vi "KWP Diagnostics Engine.vi"(8 "error in (no error)":errorcluster, 11 "State Variables":T1={"TCP Refs"={"Connection List"=refnum, "listener ID"=refnum}, "Stop"=refnum, "Top VI"=refnum, "Parameters"={"Name"="", "PID Lookup"=variant, "DID Lookup"=variant, "Section Properties"={"CAN"={"Database File"=path "", "CAN Interface"=enum."CAN0", "Baud Rate"=0, "Diagnostic Protocol"=enum."GMLAN", "Transport Protocol"=enum."ISO TP - Normal Mode", "Transmit ID"=0, "Receive ID"=0, "Transmit Extension"=0, "Receive Extension"=0, "Receive UUDT ID"=0, "Enable Stream"=TRUE, "VW TP Channel ID"=0}, "DPIDs"=[], "DTC descriptor"={"DTC Byte Length"=2, "Status Byte Length"=1, "Add Data Byte Length"=1, "Byte Order"=enum."Motorola"}, "PIDs"=[], "DIDs"=[], "CPIDs"=[]}, "ChanRefs"={"ToVS.PIDs"={"Name"="", "Write to VS Engine FIFO"=refnum, "Pairs"={"Refs"=[], "Values"=[]}}, "ToVS.DIDs"={"Name"="", "Write to VS Engine FIFO"=refnum, "Pairs"={"Refs"=[], "Values"=[]}}, "ToVS.DTCs"={"Name"="", "Write to VS Engine FIFO"=refnum, "Pairs"={"Refs"=[], "Values"=[]}}, "ToVS.DTCCount"={"Name"="", "Write to VS Engine FIFO"=refnum, "Pairs"={"Refs"=[], "Values"=[]}}, "ToVS.Success"={"Name"="", "Write to VS Engine FIFO"=refnum, "Pairs"={"Refs"=[], "Values"=[]}}, "FromVS.CPIDs"={"Name"="", "Read from VS Engine FIFO"=refnum, "Pairs"={"Refs"=[], "Values"=[]}}, "Cmds"={"Name"="", "Write to VS Engine FIFO"=refnum, "Read from VS Engine FIFO"=refnum, "Pairs"={"Chan Refs"=[], "Prev. Values"=[]}}}, "CPID Lookup"=variant, "DPID Lookup"=variant}, "ADCS Connection"={"Diag CAN Handle"=0, "Transport Protocol"=enum."ISO TP - Normal Mode", "Receive Address Extension"=0, "Transmit Address Extension"=0, "Receive CAN Id"=0, "Transmit CAN Id"=0, "Diag CAN Queue"=refnum, "Log Frames ?"=FALSE, "My TP Address"=0, "Other TP Address"=0, "T1"=0, "T2"=0, "T3"=0, "T4"=0, "Tx SN"=0, "Block Size"=0, "Rx SN"=0, "VW TP Initialized?"=FALSE, "Tx block no"=0, "baud rate"=0, "Interface"="", "Channel Diag CAN Handle"=0, "UDP Connection ID"=refnum, "TCP Connection ID"=refnum, "Target IP Addr"=0, "Source Address"=0, "Target Address"=0, "Send Header NACK?"=FALSE, "DLL Handle"=0, "NAD"=0, "Time Stamp read first"=0.0, "Time Stamp read last"=0.0, "Time Stamp write first"=0.0, "Time Stamp write last"=0.0, "Time Stamp write"=0.0, "Time Stamp read"=0.0}, "XNET References"={"Database"="", "GMLAN DPID Session"="", "Cluster"=""}, "BufferedCmds"=refnum, "XNETEngine (GMLAN)"=refnum} {"Parameters"."ChanRefs"."Cmds"."Pairs"."Chan Refs" format="%.0x"; "Parameters"."ChanRefs"."ToVS.Success"."Pairs"."Refs" format="%.0x"; "Parameters"."ChanRefs"."ToVS.DTCCount"."Pairs"."Refs" format="%.0x"; "Parameters"."ChanRefs"."ToVS.DTCs"."Pairs"."Refs" format="%.0x"; "Parameters"."ChanRefs"."ToVS.PIDs"."Pairs"."Refs" format="%.0x"; "Parameters"."ChanRefs"."ToVS.DIDs"."Pairs"."Refs" format="%.0x"; "Parameters"."Section Properties"."CPIDs"."Signals"."Byte Order" items=["Little Endian", "Big Endian"]; "Parameters"."Section Properties"."CPIDs"."Signals"."Data Type" items=["Signed", "Unsigned", "IEEE Float"]; "Parameters"."Section Properties"."DIDs"."Signals"."Byte Order" items=["Little Endian", "Big Endian"]; "Parameters"."Section Properties"."DIDs"."Signals"."Data Type" items=["Signed", "Unsigned", "IEEE Float"]; "Parameters"."Section Properties"."CAN"."VW TP Channel ID" format="%.0x"; "Parameters"."Section Properties"."CAN"."Receive UUDT ID" format="%.0x"; "Parameters"."Section Properties"."CAN"."Receive Extension" format="%.0x"; "Parameters"."Section Properties"."CAN"."Transmit Extension" format="%.0x"; "Parameters"."Section Properties"."CAN"."Receive ID" format="%.0x"; "Parameters"."Section Properties"."CAN"."Transmit ID" format="%.0x"; "Parameters"."Section Properties"."PIDs"."Signals"."Byte Order" items=["Little Endian", "Big Endian"]; "Parameters"."Section Properties"."PIDs"."Signals"."Data Type" items=["Signed", "Unsigned", "IEEE Float"]}) -> (0 "error out":errorcluster)   [LabVIEW 2015, in "Diagnostics Addon Engine.lvlib"]
uses:
  Diagnostics Addon Engine.lvlib
  State Variables.ctl
  TCP Refs.ctl
  STM/STM Lookup Table Ref.ctl
  Stop FG/Stop Global Ref.ctl
  Main Configuration.ctl
  Section Properties.ctl
  Shared/CAN Configuration.ctl
  Shared/CAN Interface.ctl
  Shared/Diagnostic Protocols.ctl
  Shared/Transport Protocols.ctl
  Shared/DPID Parameters.ctl
  Shared/DPID Periodic Rate.ctl
  <vilib>/Automotive Diagnostic Command Set/Diagnostic Protocols.llb/DTC Descriptor.ctl
  Shared/DIDPID Parameters.ctl
  Shared/DIDPID Signal Parameters.ctl
  VS Data Channels.ctl
  Inline Async API/Controls/Write To VS Engine.ctl
  <vilib>/NI Veristand/Custom Device API/Data Reference.ctl
  Inline Async API/Controls/Read From VS Engine.ctl
  <vilib>/NI Veristand/Custom Device API/Block Data Reference.ctl
  Inline Async API/Controls/ReadWrite Data.ctl
  <vilib>/Automotive Diagnostic Command Set/Diagnostic Transport.llb/Diag Reference.ctl
  <vilib>/Automotive Diagnostic Command Set/Diagnostic Transport.llb/Transport Protocol Selector.ctl
  <vilib>/Automotive Diagnostic Command Set/Diagnostic Transport.llb/Diag CAN Frame Log.ctl
  XNET References.ctl
  <vilib>/NI/AMC/Message Queue.ctl
  <vilib>/NI/AMC/Message.ctl
  <vilib>/NI/Tools/Keyed Array/KeyedArray.ctl
  Stop FG/Stop Global Commands.ctl
  Shared/DTC and Timestamp Cluster.ctl
  Datatable Lookup Positions.ctl
  <vilib>/NI/AMC/Create Single Message.vi
  <vilib>/NI/AMC/Update Message Routing Info.vi
  <vilib>/NI/Tools/Keyed Array/Map String.vi
  <vilib>/NI/AMC/Read Termination Message.vi
  <vilib>/NI/Tools/String/Get Case Matching.vi
  <vilib>/xnet/xnet.llb/XNET Convert (Frame Raw to Signal).vi
  Convert ID to Raw Data.vi
  Shared/GUID Lookup.vi
  <vilib>/NI/AMC/Send Message.vi
  <vilib>/NI/AMC/Globals.vi
  Stop FG/Stop FG.lvlib
  Error Handling API/Error Handling API.lvlib
  <vilib>/NI Veristand/Custom Device Tools/Custom Device Utility Library/Custom Device Utility Library.lvlib
  Shared/Diagnostics Addon Shared.lvlib
  <vilib>/NI/AMC/AMC.lvlib
  <vilib>/NI/Tools/Keyed Array/Tools_KeyedArray.lvlib
  <vilib>/NI Veristand/Custom Device API/Custom Device API.lvlib
  <vilib>/addons/Automotive Diagnostic Command Set/NI_Automotive Diagnostic Command Set.lvlib
  Inline Async API/Inline Async API.lvlib
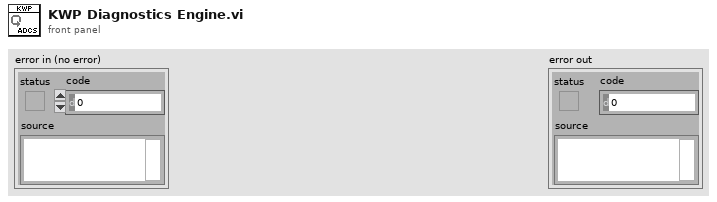
[diagram p1: front panel]
types:
  T1 = typedef "Diagnostics Addon Engine.lvlib/State Variables.ctl" = cluster{"TCP Refs":T2, "Stop":T4, "Top VI":refnum<vi>, "Parameters":T5, "ADCS Connection":T22, "XNET References":T24, "BufferedCmds":T25, "XNETEngine (GMLAN)":T25}
  T2 = typedef "Diagnostics Addon Engine.lvlib/TCP Refs.ctl" = cluster{"Connection List":T3, "listener ID":refnum<k5>}
  T3 = typedef "Diagnostics Addon Engine.lvlib/STM Lookup Table Ref.ctl" = refnum<vi>
  T4 = typedef "Diagnostics Addon Engine.lvlib/Stop FG.lvlib/Stop Global Ref.ctl" = refnum<vi>
  T5 = typedef "Diagnostics Addon Engine.lvlib/Main Configuration.ctl" = cluster{"Name":string, "PID Lookup":variant, "DID Lookup":variant, "Section Properties":T6, "ChanRefs":T16, "CPID Lookup":variant, "DPID Lookup":variant}
  T6 = typedef "Diagnostics Addon Engine.lvlib/Section Properties.ctl" = cluster{"CAN":T7, "DPIDs":T11[], "DTC descriptor":T13, "PIDs":T14[], "DIDs":T14[], "CPIDs":T14[]}
  T7 = typedef "Diagnostics Addon Shared.lvlib/CAN Configuration.ctl" = cluster{"Database File":path, "CAN Interface":T8, "Baud Rate":u32, "Diagnostic Protocol":T9, "Transport Protocol":T10, "Transmit ID":u32, "Receive ID":u32, "Transmit Extension":u8, "Receive Extension":u8, "Receive UUDT ID":u32, "Enable Stream":bool, "VW TP Channel ID":u32}
  T8 = typedef "Diagnostics Addon Shared.lvlib/CAN Interface.ctl" = enum16{"CAN0", "CAN1", "CAN2", "CAN3", "CAN4", "CAN5", "CAN6", "CAN7", "CAN8", "CAN9", "CAN10", "CAN11", "CAN12", "CAN13", "CAN14", "CAN15", "CAN16", "CAN17", "CAN18", "CAN19", "CAN20", "CAN21", "CAN22", "CAN23", "CAN24", "CAN25", "CAN26", "CAN27", "CAN28", "CAN29", "CAN30", "CAN31", "CAN32", "CAN33", "CAN34", "CAN35", "CAN36", "CAN37", "CAN38", "CAN39", "CAN40", "CAN41", "CAN42", "CAN43", "CAN44", "CAN45", "CAN46", "CAN47", "CAN48", "CAN49", "CAN50", "CAN51", "CAN52", "CAN53", "CAN54", "CAN55", "CAN56", "CAN57", "CAN58", "CAN59", "CAN60", "CAN61", "CAN62", "CAN63", "CAN 256 (Virtual)", "CAN 257 (Virtual)"}
  T9 = typedef "Diagnostics Addon Shared.lvlib/Diagnostic Protocols.ctl" = enum16{"GMLAN", "KWP-2000", "UDS"}
  T10 = typedef "Diagnostics Addon Shared.lvlib/Transport Protocols.ctl" = enum16{"ISO TP - Normal Mode", "ISO TP - Mixed Mode", "VW TP 2.0", "Diagnostics on IP"}
  T11 = typedef "Diagnostics Addon Shared.lvlib/DPID Parameters.ctl" = cluster{"DPID ID":u8, "Speed":T12, "PIDs":u16[]}
  T12 = typedef "Diagnostics Addon Shared.lvlib/DPID Periodic Rate.ctl" = enum16{"Slow", "Medium", "Fast"}
  T13 = typedef "DTC Descriptor.ctl" = cluster{"DTC Byte Length":i32, "Status Byte Length":i32, "Add Data Byte Length":i32, "Byte Order":enum16{"Motorola", "Intel"}}
  T14 = typedef "Diagnostics Addon Shared.lvlib/DIDPID Parameters.ctl" = cluster{"Name":string, "Description":string, "ID":u16, "Signals":T15[]}
  T15 = typedef "Diagnostics Addon Shared.lvlib/DIDPID Signal Parameters.ctl" = cluster{"Start Bit":u8, "Length":u8, "Scaling Factor":dbl, "Scaling Offset":dbl, "Minimum":dbl, "Maximum":dbl, "Data Type":u32, "Byte Order":u32, "Default Value":dbl, "Name":string, "Units":string, "Description":string}
  T16 = typedef "Diagnostics Addon Engine.lvlib/VS Data Channels.ctl" = cluster{"ToVS.PIDs":T17, "ToVS.DIDs":T17, "ToVS.DTCs":T17, "ToVS.DTCCount":T17, "ToVS.Success":T17, "FromVS.CPIDs":T19, "Cmds":T21}
  T17 = typedef "Diagnostics Addon Engine.lvlib/Inline Async API.lvlib/Write To VS Engine.ctl" = cluster{"Name":string, "Write to VS Engine FIFO":refnum<k33>, "Pairs":cluster{"Refs":T18[], "Values":dbl[]}}
  T18 = typedef "Custom Device API.lvlib/Data Reference.ctl" = i32
  T19 = typedef "Diagnostics Addon Engine.lvlib/Inline Async API.lvlib/Read From VS Engine.ctl" = cluster{"Name":string, "Read from VS Engine FIFO":refnum<k33>, "Pairs":cluster{"Refs":T20[], "Values":dbl[]}}
  T20 = typedef "Custom Device API.lvlib/Block Data Reference.ctl" = cluster{"Data Reference":T18, "Offset":u64, "Length":u64}
  T21 = typedef "Diagnostics Addon Engine.lvlib/Inline Async API.lvlib/ReadWrite Data.ctl" = cluster{"Name":string, "Write to VS Engine FIFO":refnum<k33>, "Read from VS Engine FIFO":refnum<k33>, "Pairs":cluster{"Chan Refs":T18[], "Prev. Values":dbl[]}}
  T22 = typedef "NI_Automotive Diagnostic Command Set.lvlib/Diag Reference.ctl" = cluster{"Diag CAN Handle":u32, "Transport Protocol":T23, "Receive Address Extension":u8, "Transmit Address Extension":u8, "Receive CAN Id":u32, "Transmit CAN Id":u32, "Diag CAN Queue":refnum<queue>, "Log Frames ?":bool, "My TP Address":u8, "Other TP Address":u8, "T1":u16, "T2":u16, "T3":u16, "T4":u16, "Tx SN":u8, "Block Size":u8, "Rx SN":u8, "VW TP Initialized?":bool, "Tx block no":u8, "baud rate":u32, "Interface":string, "Channel Diag CAN Handle":u32, "UDP Connection ID":refnum<k16>, "TCP Connection ID":refnum<k5>, "Target IP Addr":u32, "Source Address":u16, "Target Address":u16, "Send Header NACK?":bool, "DLL Handle":u32, "NAD":u8, "Time Stamp read first":dbl, "Time Stamp read last":dbl, "Time Stamp write first":dbl, "Time Stamp write last":dbl, "Time Stamp write":dbl, "Time Stamp read":dbl}
  T23 = typedef "NI_Automotive Diagnostic Command Set.lvlib/Transport Protocol Selector.ctl" = enum16{"ISO TP - Normal Mode", "ISO TP - Mixed Mode", "VW TP 2.0", "Diagnostics on IP", "ISO TP LIN"}
  T24 = typedef "Diagnostics Addon Engine.lvlib/XNET References.ctl" = cluster{"Database":refnum<k21>, "GMLAN DPID Session":refnum<k21>, "Cluster":refnum<k21>}
  T25 = typedef "AMC.lvlib/Message Queue.ctl" = refnum<queue>
  T26 = typedef "Diagnostics Addon Shared.lvlib/DTC and Timestamp Cluster.ctl" = cluster{"Timestamp":dbl, "DTC":dbl, "Status":dbl, "Add Data":dbl}
  T27 = typedef "Diagnostics Addon Engine.lvlib/Stop FG.lvlib/Stop Global Commands.ctl" = enum16{"Write", "Read", "Reset"}
  T28 = typedef "Diagnostics Addon Engine.lvlib/Datatable Lookup Positions.ctl" = cluster{"Offset":i32, "Length":i32}
  T29 = typedef "AMC.lvlib/Message.ctl" = cluster{"name":string, "value":string, "attributes":T30, "receiver host":string, "receiver process":string, "source host":string, "source process":string, "priority message":bool, "acknowledge message":bool}
  T30 = typedef "Tools_KeyedArray.lvlib/KeyedArray.ctl" = cluster{"keys":string[], "values":string[]}
  T31 = typedef "Diagnostic Trouble Code.ctl" = cluster{"DTC":u32, "Status":u32, "Add Data":u32}
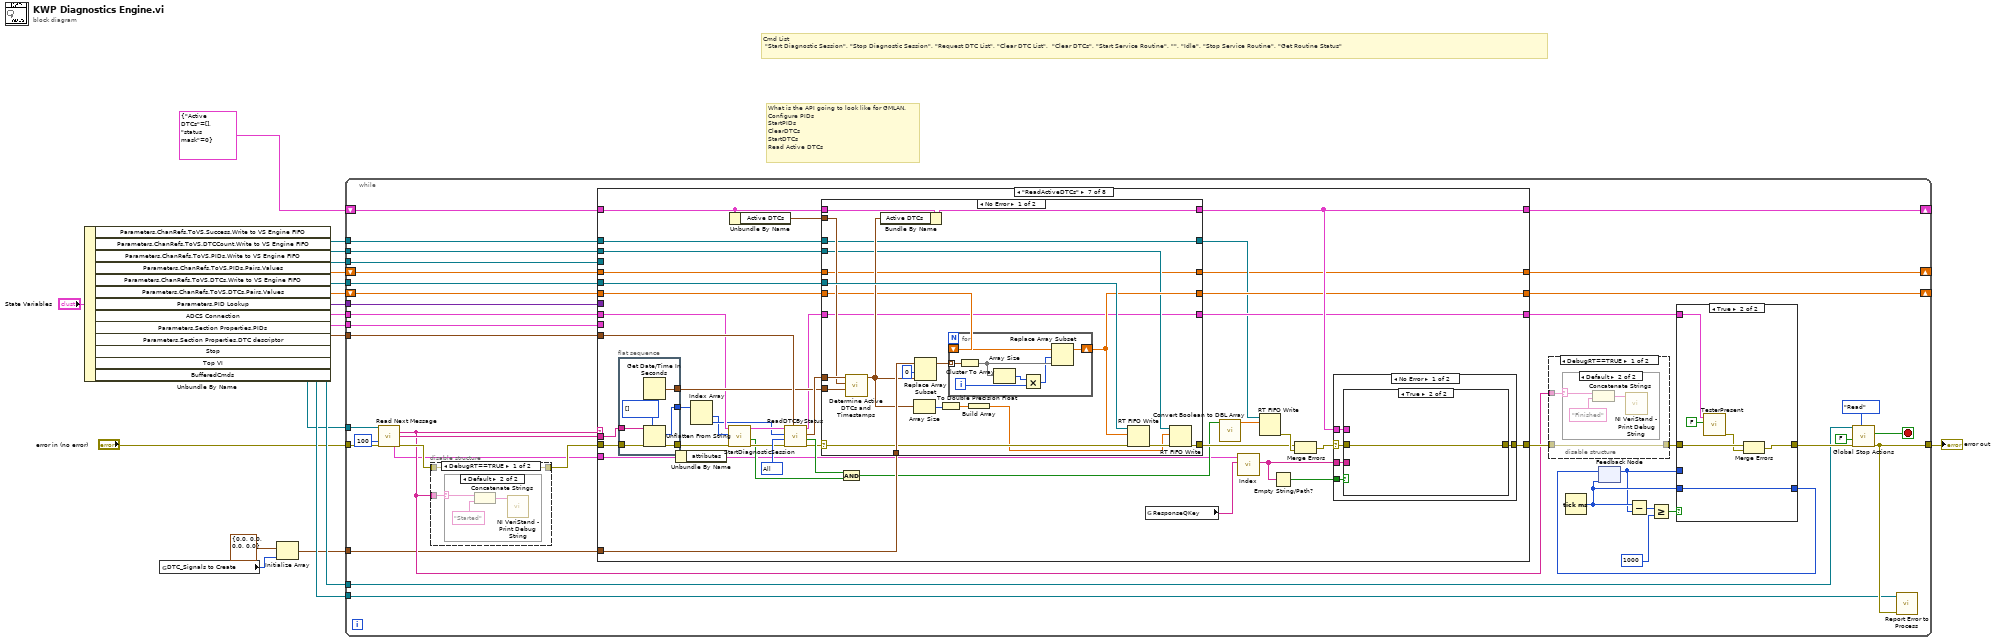
[diagram p0: block diagram]
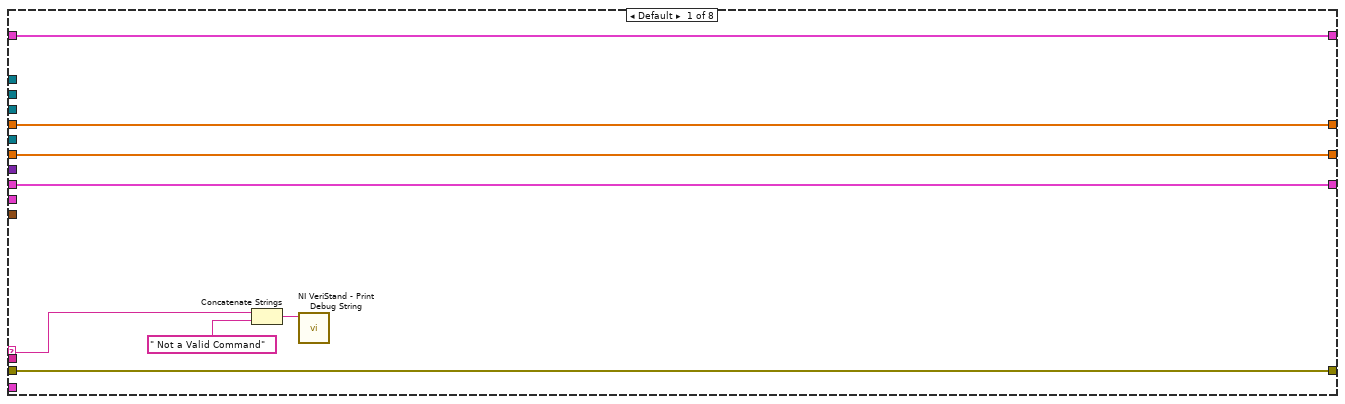
[diagram p7: hidden frame]
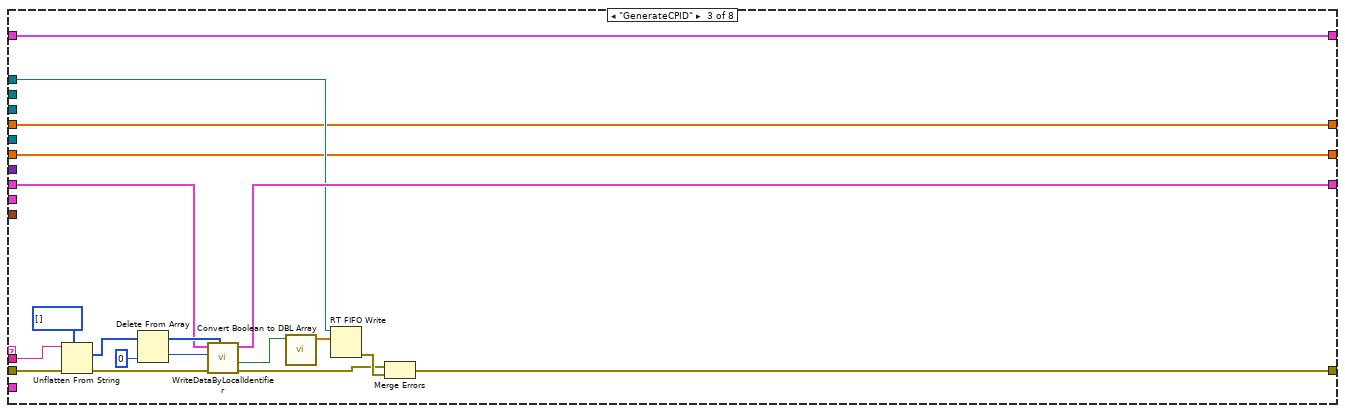
[diagram p9: hidden frame]
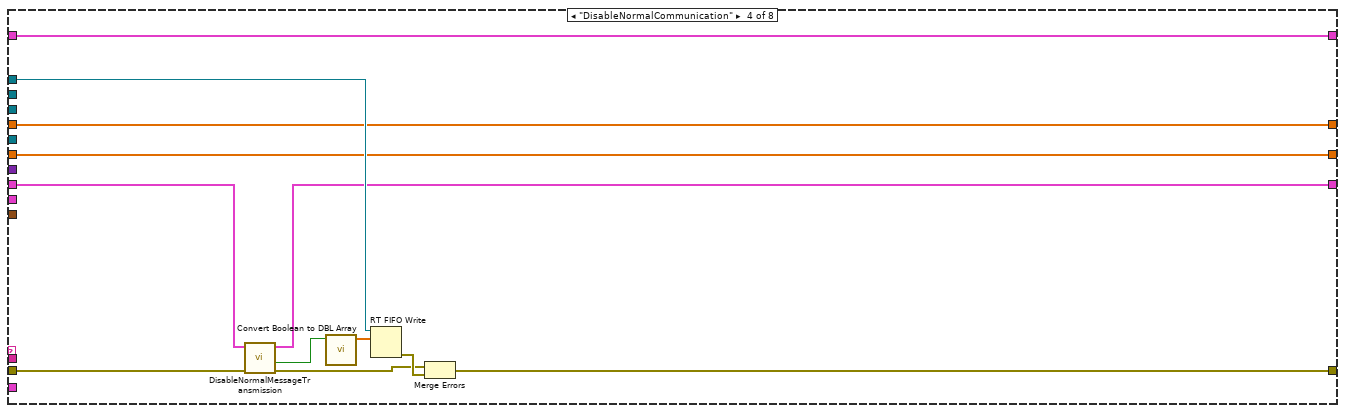
[diagram p10: hidden frame]
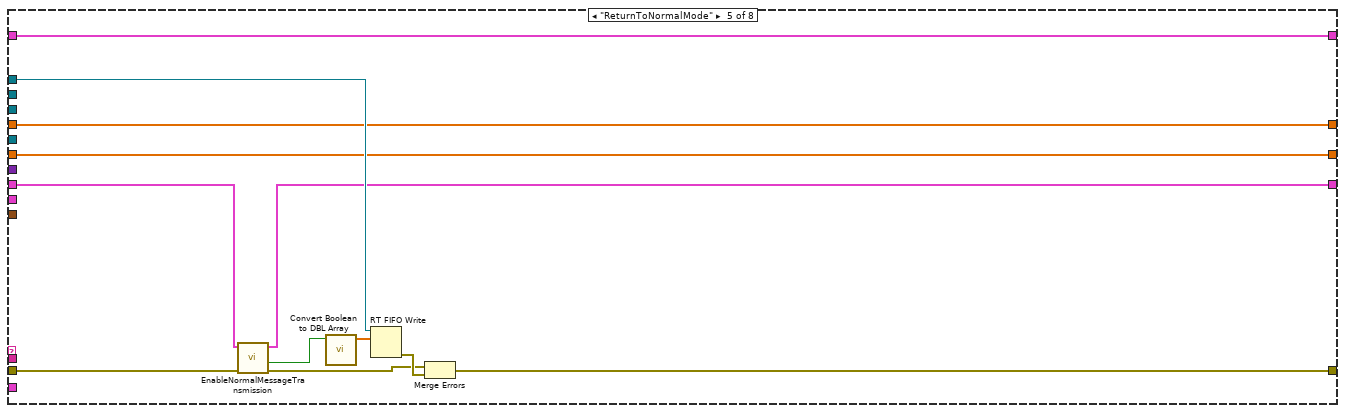
[diagram p11: hidden frame]
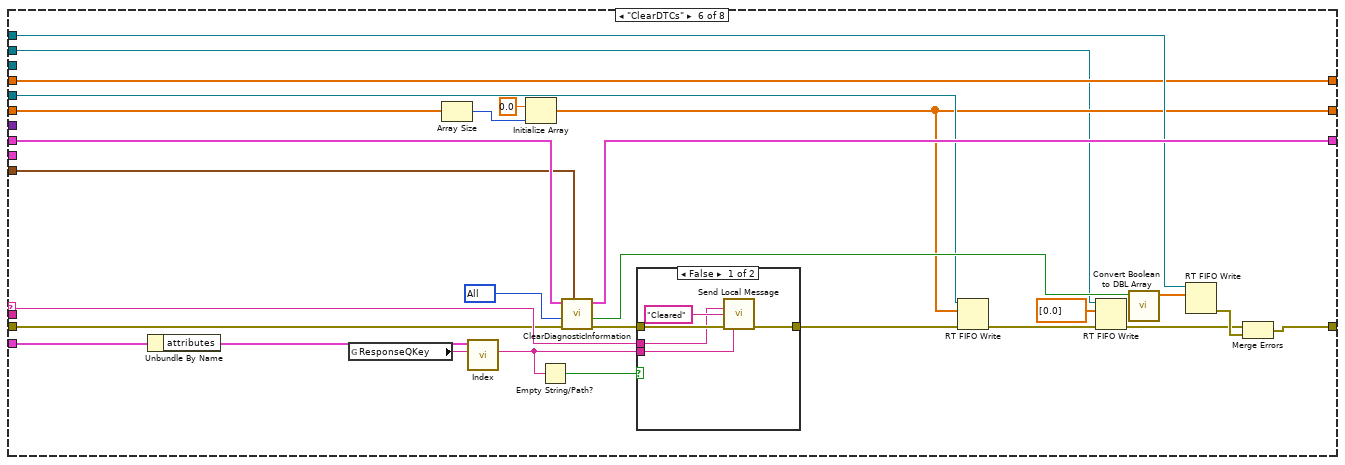
[diagram p12: hidden frame]
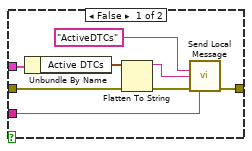
[diagram p14: hidden frame]
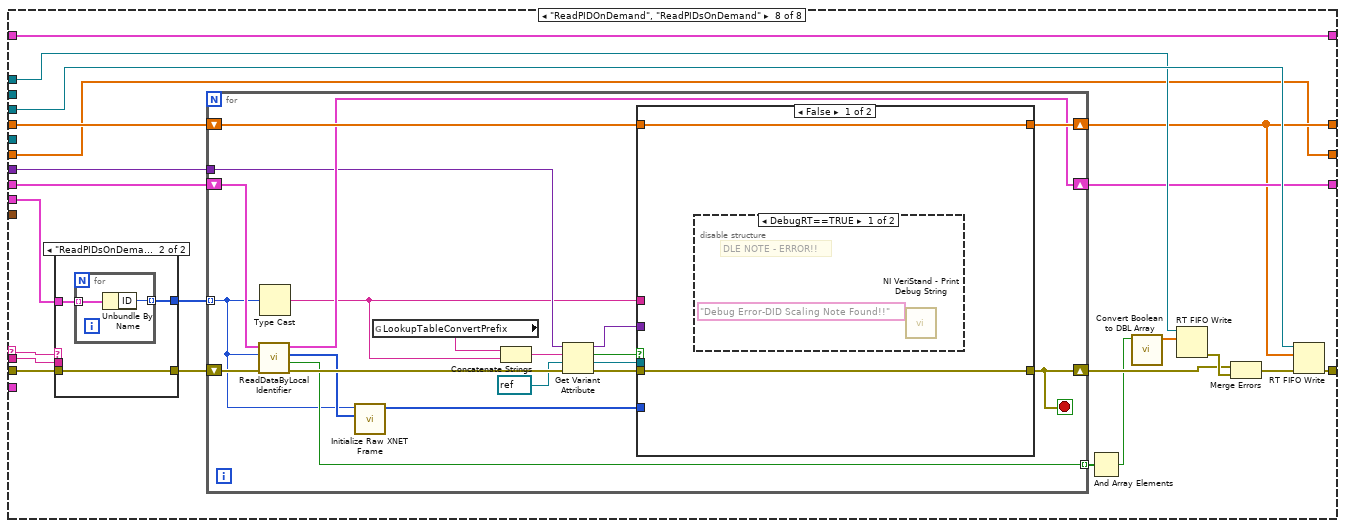
[diagram p17: hidden frame]
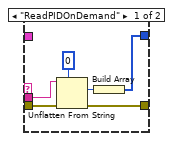
[diagram p18: hidden frame]
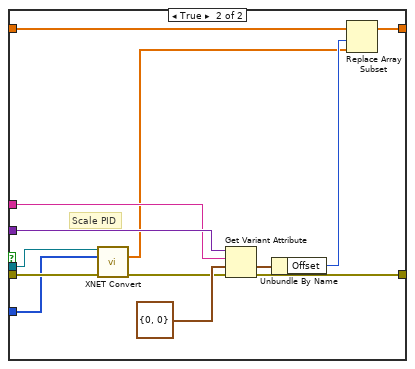
[diagram p20: hidden frame]
diagram:
  # "What is the API going to look like for GMLAN.\nConfigure PIDs\nStartPIDs\nClearDTCs\nStartDTCs\nRead Active DTCs"
  # "Cmd List\n \"Start Diagnostic Session\", \"Stop Diagnostic Session\", \"Request DTC List\", \"Clear DTC List\",  \"Clear DTCs\", \"Start Service Routine\", \"\", \"Idle\", \"Stop Service Routine\", \"Get Routine Status\""
  n1 = Unbundle By Name("State Variables") -> ("Parameters.ChanRefs.ToVS.Success.Write to VS Engine FIFO"=w13:refnum<k33>, "Parameters.ChanRefs.ToVS.DTCCount.Write to VS Engine FIFO"=w1:refnum<k33>, "Parameters.ChanRefs.ToVS.PIDs.Write to VS Engine FIFO"=w2:refnum<k33>, "Parameters.ChanRefs.ToVS.PIDs.Pairs.Values"=w7:dbl[], "Parameters.ChanRefs.ToVS.DTCs.Write to VS Engine FIFO"=w8:refnum<k33>, "Parameters.ChanRefs.ToVS.DTCs.Pairs.Values"=w9:dbl[], "Parameters.PID Lookup"=w19:variant, "ADCS Connection"=w15:T22, "Parameters.Section Properties.PIDs"=w11:T14[], "Parameters.Section Properties.DTC descriptor"=w6:T13, "Stop"=w20:T4, "Top VI"=w17:refnum<vi>, "BufferedCmds"=w10:T25)
  n2 = global read "GUID Lookup.vi" "DTC_Signals to Create"() -> (w4:i32)
  n3 = Initialize Array(T26 {"Timestamp"=0.0, "DTC"=0.0, "Status"=0.0, "Add Data"=0.0} ("Diagnostic Trouble Code"), w4) -> (w3:T26[])
  n4 = while {
    tunnel: w10 -> [w59]
    tunnel: w15 -> [w53]
    tunnel: w17 -> [w42]
    tunnel: "error in (no error)" -> [w57]
    tunnel: [w44] -> w16
    tunnel: w19 -> [w41]
    tunnel: w20 -> [w40]
    shift-right: [w39] -> _
    shift-left: cluster{"Active DTCs":T26[], "status mask":u8} {"Active DTCs"=[], "status mask"=0} -> [w38]
    tunnel: w13 -> [w31]
    tunnel: w11 -> [w30]
    tunnel: w8 -> [w28]
    tunnel: w2 -> [w26]
    shift-right: [w25] -> _
    shift-left: w7 -> [w27]
    shift-right: [w24] -> _
    shift-left: w9 -> [w29]
    tunnel: w6 -> [w23]
    tunnel: w3 -> [w22]
    tunnel: w1 -> [w21]
    stop <- w43 stop-if-true
    n5 = call <vilib>:"Read Next Message.vi"("message queue in"=w59, "timeout (1 ms)"=100 ("timeout (1ms)"), "error in"=w57) -> ("message name"=w33:string, "message value"=w54:string, "message"=w32:T29, "error out"=w35:errorcluster)  [unwired: 5 in, 4 out]
    n6 = disable-structure shown="DebugRT==TRUE" {
      disable-tunnel: w33 -> [w61 _]
      disable-tunnel: [w60 w65] -> w34
      disable-tunnel: w35 -> [w60 w65]
      frame condition #0 {
        n7 = case shown="Default" w61 {
          selector: w61 -> [_ w62]
          frame "" {
          }
          frame Default {
            n8 = Concatenate Strings(w62, "Started" ("string")) -> (w64:string)
            n9 = call <vilib>:"NI VeriStand - Print Debug String.vi"("Message"=w64) -> ()  [unwired: 10 in, 1 out]
          }
        }
      }
      frame condition #1 (active) {
      }
    }
    n10 = case shown="\"ReadActiveDTCs\"" w33 {
      selector: w33 -> [w82 _ _ _ _ w158 _ w277]
      tunnel: w34 -> [w86 w91 w110 w116 w130 w142 w196 w279]
      tunnel: w54 -> [_ _ w109 _ _ _ w195 w278]
      tunnel: [w86 w91 w97 w120 w132 w153 w210 w267] -> w36
      tunnel: w53 -> [w87 w92 w103 w118 w128 w163 w184 w275]
      tunnel: [w87 w92 w102 w117 w127 w162 w177 w270] -> w48
      tunnel: w41 -> [_ _ _ _ _ _ _ w274]
      tunnel: [w85 w90 w111 w123 w135 _ w197 w288] -> w39
      tunnel: w38 -> [w85 w90 w111 w123 w135 _ w198 w288]
      tunnel: w32 -> [_ _ _ _ _ w160 w209 _]
      tunnel: w31 -> [_ _ w95 w119 w131 w155 w175 w271]
      tunnel: w30 -> [_ _ _ _ _ _ _ w276]
      tunnel: w29 -> [w80 w88 w93 w112 w124 w147 w193 w268]
      tunnel: w28 -> [_ _ _ _ _ w150 w202 _]
      tunnel: w27 -> [w81 w89 w94 w113 w125 w152 w173 w273]
      tunnel: w26 -> [_ _ _ _ _ _ _ w272]
      tunnel: [w81 w89 w94 w113 w125 w152 w172 w269] -> w25
      tunnel: [w80 w88 w93 w112 w124 w146 w192 w268] -> w24
      tunnel: w23 -> [_ _ _ _ _ w145 w207 _]
      tunnel: w22 -> [_ _ _ _ _ _ w194 _]
      tunnel: w21 -> [_ _ _ _ _ w139 w190 _]
      frame Default {
        n11 = Concatenate Strings(w82, " Not a Valid Command" ("string")) -> (w83:string)
        n12 = call <vilib>:"NI VeriStand - Print Debug String.vi"("Message"=w83) -> ()  [unwired: 10 in, 1 out]
      }
      frame "" {
      }
      frame "GenerateCPID" {
        n13 = Unflatten From String(type=u8[] [], binary string=w109, error in (no error)=w110) -> (value=w107:u8[], error out=w101:errorcluster)  [unwired: 2 in, 1 out]
        n14 = Delete From Array(array=w107, index=0) -> (deleted portion=w105:u8, array with subset deleted=w104:u8[])  [unwired: 1 in]
        n15 = call <vilib>:"WriteDataByLocalIdentifier.vi"("data in"=w104, "error in (no error)"=w101, "local ID"=w105, "diag ref in"=w103) -> ("error out"=w98:errorcluster, "success?"=w96:bool, "diag ref out"=w102:T22)  [unwired: 5 in]
        n16 = call "Convert Boolean to DBL Array.vi"("Boolean"=w96) -> ("DBL Array"=w100:dbl[])  [unwired: 10 in]
        n17 = RT FIFO Write(0:w95, 1:w100) -> (11:w99:errorcluster)  [unwired: 3 in, 3 out]
        n18 = Merge Errors(w98, w99) -> (w97:errorcluster)
      }
      frame "DisableNormalCommunication" {
        n19 = call <vilib>:"DisableNormalMessageTransmission.vi"("error in (no error)"=w116, "diag ref in"=w118) -> ("error out"=w115:errorcluster, "success?"=w114:bool, "diag ref out"=w117:T22)  [unwired: 7 in]
        n20 = call "Convert Boolean to DBL Array.vi"("Boolean"=w114) -> ("DBL Array"=w122:dbl[])  [unwired: 10 in]
        n21 = RT FIFO Write(0:w119, 1:w122) -> (11:w121:errorcluster)  [unwired: 3 in, 3 out]
        n22 = Merge Errors(w115, w121) -> (w120:errorcluster)
      }
      frame "ReturnToNormalMode" {
        n23 = call <vilib>:"EnableNormalMessageTransmission.vi"("error in (no error)"=w130, "diag ref in"=w128) -> ("error out"=w129:errorcluster, "success?"=w126:bool, "diag ref out"=w127:T22)  [unwired: 7 in]
        n24 = call "Convert Boolean to DBL Array.vi"("Boolean"=w126) -> ("DBL Array"=w134:dbl[])  [unwired: 10 in]
        n25 = RT FIFO Write(0:w131, 1:w134) -> (11:w133:errorcluster)  [unwired: 3 in, 3 out]
        n26 = Merge Errors(w129, w133) -> (w132:errorcluster)
      }
      frame "ClearDTCs" {
        w141 = u16 65280 items=["Powertrain"=0, "Chassis"=16384, "Body"=32768, "Network"=49152, "All"=65280] ("Group of DTC")
        n27 = Unbundle By Name(w160) -> ("attributes"=w136:T30)
        n28 = global read "GUID Lookup.vi" "ResponseQKey"() -> (w159:string)
        n29 = Array Size(array=w147) -> (size(s)=w149:i32)
        n30 = call <vilib>:"Index.vi"("key"=w159, "array in"=w136) -> ("value"=w144:string)  [unwired: 3 in, 2 out]
        n31 = Initialize Array(0.0 ("element"), w149) -> (w146:dbl[])
        n32 = Empty String/Path?(string/path=w144) -> (empty?=w143:bool)
        n33 = call <vilib>:"ClearDiagnosticInformation.vi"("DTC descriptor"=w145, "error in (no error)"=w142, "group of DTC"=w141, "diag ref in"=w163) -> ("error out"=w161:errorcluster, "success?"=w156:bool, "diag ref out"=w162:T22)  [unwired: 5 in]
        n34 = case shown="False" w143 {
          tunnel: w161 -> [w168 w169]
          tunnel: [w167 w169] -> w151
          tunnel: w144 -> [w165 _]
          tunnel: w158 -> [w164 _]
          frame False {
            n35 = call <vilib>:"Send Local Message.vi"("receiver process (\"\" - local)"=w165, "message name"=w164, "message value"="Cleared" ("Message Value"), "error in"=w168) -> ("error out"=w167:errorcluster)  [unwired: 9 in, 2 out]
          }
          frame True {
          }
        }
        n36 = RT FIFO Write(0:w150, 1:w146, 3:w151) -> (11:w138:errorcluster)  [unwired: 2 in, 3 out]
        n37 = RT FIFO Write(0:w139, 1:dbl[] [0.0] ("element"), 3:w138) -> (11:w137:errorcluster)  [unwired: 2 in, 3 out]
        n38 = call "Convert Boolean to DBL Array.vi"("Boolean"=w156) -> ("DBL Array"=w157:dbl[])  [unwired: 10 in]
        n39 = RT FIFO Write(0:w155, 1:w157) -> (11:w154:errorcluster)  [unwired: 3 in, 3 out]
        n40 = Merge Errors(w137, w154) -> (w153:errorcluster)
      }
      frame "ReadActiveDTCs" {
        w188 = u16 65280 items=["Powertrain"=0, "Chassis"=16384, "Body"=32768, "Network"=49152, "All"=65280] ("Group of DTC")
        n41 = flat-sequence {
          tunnel: [w266] -> w200
          tunnel: [w264] -> w187
          tunnel: w196 -> [w265]
          tunnel: w195 -> [w263]
          tunnel: [w262] -> w181
          frame #0 {
            n42 = Get Date/Time In Seconds() -> (seconds since 1Jan1904=w266:timestamp)
            n43 = Unflatten From String(type=u8[] [], binary string=w263, error in (no error)=w265) -> (value=w262:u8[], error out=w264:errorcluster)  [unwired: 2 in, 1 out]
          }
        }
        n44 = Unbundle By Name(w209) -> ("attributes"=w170:T30)
        n45 = Index Array(array=w181) -> (element #1=w179:u8, element #2=w180:u8)  [unwired: 2 in]
        n46 = call <vilib>:"StartDiagnosticSession.vi"("error in (no error)"=w187, "mode"=w179, "diag ref in"=w184) -> ("error out"=w186:errorcluster, "success?"=w182:bool, "diag ref out"=w185:T22)  [unwired: 6 in]
        n47 = Unbundle By Name(w198) -> ("Active DTCs"=w199:T26[])
        n48 = call <vilib>:"ReadDTCByStatus.vi"("DTC descriptor"=w207, "error in (no error)"=w186, "group of DTC"=w188, "mode"=w180, "diag ref in"=w185) -> ("error out"=w178:errorcluster, "success?"=w189:bool, "DTCs"=w201:T31[], "diag ref out"=w176:T22)  [unwired: 3 in]
        n49 = case shown="No Error" w178 {
          selector: w178 -> [w230 w258]
          tunnel: w202 -> [w247 _]
          tunnel: w201 -> [w246 _]
          tunnel: w200 -> [w245 _]
          tunnel: w199 -> [w244 _]
          tunnel: w198 -> [w243 w259]
          tunnel: [w242 w259] -> w197
          tunnel: w194 -> [w237 _]
          tunnel: w193 -> [w235 w260]
          tunnel: [w234 w260] -> w192
          tunnel: [w232 w258] -> w191
          tunnel: w190 -> [w231 _]
          tunnel: [w228 w257] -> w177
          tunnel: w176 -> [w228 w257]
          tunnel: w175 -> [w227 w256]
          tunnel: [w227 w256] -> w174
          tunnel: w173 -> [w226 w255]
          tunnel: [w226 w255] -> w172
          frame No Error {
            n50 = call "Determine Active DTCs and Timestamps.vi"("current Time Stamp"=w245, "Previous Changed DTCs"=w244, "current DTCs"=w246) -> ("Active DTCs"=w236:T26[])  [unwired: 8 in]
            n51 = Bundle By Name(cluster=w243, "Active DTCs"=w236) -> (w242:cluster{"Active DTCs":T26[], "status mask":u8})
            n52 = Array Size(array=w236) -> (size(s)=w240:i32)
            n53 = Replace Array Subset(array=w237, new element=w236, index=0) -> (w239:T26[])
            n54 = To Double Precision Float(number=w240) -> (double precision float=w241:dbl)
            n55 = for {
              tunnel: w239 -> [w254] mode=indexing
              shift-right: [w253] -> w234
              shift-left: w235 -> [w252]
              i -> [w249]
              n56 = Cluster To Array(cluster=w254) -> (array=w251:dbl[])
              n57 = Array Size(array=w251) -> (size(s)=w250:i32)
              n58 = Multiply(x=w250, y=w249) -> (x*y=w248:i32)
              n59 = Replace Array Subset(array=w252, new element=w251, index=w248) -> (w253:dbl[])
            }
            n60 = Build Array(w241) -> (w229:dbl[])
            n61 = RT FIFO Write(0:w247, 1:w234, 3:w230) -> (11:w233:errorcluster)  [unwired: 2 in, 3 out]
            n62 = RT FIFO Write(0:w231, 1:w229, 3:w233) -> (11:w232:errorcluster)  [unwired: 2 in, 3 out]
          }
          frame Error {
          }
        }
        n63 = And(x=w189, y=w182) -> (x .and. y?=w183:bool)
        n64 = global read "GUID Lookup.vi" "ResponseQKey"() -> (w208:string)
        n65 = call "Convert Boolean to DBL Array.vi"("Boolean"=w183) -> ("DBL Array"=w204:dbl[])  [unwired: 10 in]
        n66 = call <vilib>:"Index.vi"("key"=w208, "array in"=w170) -> ("value"=w205:string)  [unwired: 3 in, 2 out]
        n67 = RT FIFO Write(0:w174, 1:w204) -> (11:w203:errorcluster)  [unwired: 3 in, 3 out]
        n68 = Empty String/Path?(string/path=w205) -> (empty?=w206:bool)
        n69 = Merge Errors(w191, w203) -> (w171:errorcluster)
        n70 = case shown="No Error" w171 {
          selector: w171 -> [w211 w225]
          tunnel: [w215 w225] -> w210
          tunnel: w206 -> [w214 _]
          tunnel: w205 -> [w213 _]
          tunnel: w197 -> [w212 _]
          frame No Error {
            n71 = case shown="True" w214 {
              tunnel: [w223 w224] -> w215
              tunnel: w212 -> [w219 _]
              tunnel: w211 -> [w217 w224]
              tunnel: w213 -> [w216 _]
              frame False {
                n72 = Unbundle By Name(w219) -> ("Active DTCs"=w218:T26[])
                n73 = Flatten To String(anything=w218, error in (no error)=w217) -> (data string=w220:string, error out=w221:errorcluster)  [unwired: 2 in, 1 out]
                n74 = call <vilib>:"Send Local Message.vi"("receiver process (\"\" - local)"=w216, "message name"="ActiveDTCs" ("Message Name"), "message value"=w220, "error in"=w221) -> ("error out"=w223:errorcluster)  [unwired: 9 in, 2 out]
              }
              frame True {
              }
            }
          }
          frame Error {
          }
        }
      }
      frame "ReadPIDOnDemand", "ReadPIDsOnDemand" {
        n75 = case shown="\"ReadPIDsOnDemand\", Default" w277 {
          tunnel: w276 -> [_ w297]
          tunnel: [w289 w296] -> w280
          tunnel: w279 -> [w294 w295]
          tunnel: [w293 w295] -> w281
          tunnel: w278 -> [w291 _]
          frame "ReadPIDOnDemand" {
            n76 = Unflatten From String(type=u16 0 ("ID"), binary string=w291, error in (no error)=w294) -> (value=w290:u16, error out=w293:errorcluster)  [unwired: 2 in, 1 out]
            n77 = Build Array(w290) -> (w289:u16[])
          }
          frame "ReadPIDsOnDemand", Default {
            n78 = for {
              tunnel: w297 -> [w299] mode=indexing
              tunnel: [w298] -> w296 mode=indexing
              n79 = Unbundle By Name(w299) -> ("ID"=w298:u16)
            }
          }
        }
        n80 = for {
          shift-right: [w302] -> w285
          shift-left: w281 -> [w319]
          shift-right: [w315] -> w270
          shift-left: w275 -> [w318]
          shift-right: [w316] -> w269
          shift-left: w273 -> [w317]
          tunnel: w274 -> [w313]
          tunnel: w280 -> [w300] mode=indexing
          tunnel: [w303] -> w284 mode=indexing
          stop <- w302 stop-if-true
          n81 = call <vilib>:"ReadDataByLocalIdentifier.vi"("error in (no error)"=w319, "local ID"=w300, "diag ref in"=w318) -> ("error out"=w312:errorcluster, "success?"=w303:bool, "data out"=w301:u8[], "diag ref out"=w315:T22)  [unwired: 5 in]
          n82 = Type Cast(x=w300) -> (*(type *) &x=w305:string)  [unwired: 1 in]
          n83 = call "Initialize Raw XNET Frame.vi"("Data"=w301, "identifier"=w300) -> ("Raw Frame"=w307:u8[])  [unwired: 9 in]
          n84 = global read "GUID Lookup.vi" "LookupTableConvertPrefix"() -> (w314:string)
          n85 = Concatenate Strings(w314, w305) -> (w310:string)
          n86 = Get Variant Attribute(Variant=w313, name=w310, default value (empty Variant)=refnum<k21> refnum ("DID Conversion"), error in=w312) -> (duplicate Variant=w306:variant, found=w304:bool, value=w308:refnum<k21>, error out=w311:errorcluster)
          n87 = case shown="False" w304 {
            tunnel: w317 -> [w321 w333]
            tunnel: [w321 w332] -> w316
            tunnel: [w320 w330] -> w302
            tunnel: w311 -> [w320 w329]
            tunnel: w308 -> [_ w328]
            tunnel: w307 -> [_ w327]
            tunnel: w306 -> [_ w326]
            tunnel: w305 -> [_ w325]
            frame False {
              n88 = disable-structure shown="DebugRT==TRUE" {
                frame condition #0 {
                  # "DLE NOTE - ERROR!!"
                  n89 = call <vilib>:"NI VeriStand - Print Debug String.vi"("Message"="Debug Error-DID Scaling Note Found!!" ("Debug String")) -> ()  [unwired: 10 in, 1 out]
                }
                frame condition #1 (active) {
                }
              }
            }
            frame True {
              # "Scale PID"
              n90 = call-poly <vilib>:"XNET Convert.vi"("session in"=w328, "frame data"=w327, "error in (no error)"=w329) -> ("signal data"=w323:dbl[], "error out"=w331:errorcluster)  [unwired: 10 in, 1 out]
              n91 = Get Variant Attribute(Variant=w326, name=w325, default value (empty Variant)=T28 {"Offset"=0, "Length"=0} ("cluster"), error in=w331) -> (value=w335:T28, error out=w330:errorcluster)  [unwired: 2 out]
              n92 = Unbundle By Name(w335) -> ("Offset"=w324:i32)
              n93 = Replace Array Subset(array=w333, new element=w323, index=w324) -> (w332:dbl[])
            }
          }
        }
        n94 = And Array Elements(Boolean array=w284) -> (logical AND=w282:bool)
        n95 = call "Convert Boolean to DBL Array.vi"("Boolean"=w282) -> ("DBL Array"=w283:dbl[])  [unwired: 10 in]
        n96 = RT FIFO Write(0:w271, 1:w283) -> (11:w287:errorcluster)  [unwired: 3 in, 3 out]
        n97 = Merge Errors(w285, w287) -> (w286:errorcluster)
        n98 = RT FIFO Write(0:w272, 1:w269, 3:w286) -> (11:w267:errorcluster)  [unwired: 2 in, 3 out]
      }
    }
    n99 = disable-structure shown="DebugRT==TRUE" {
      disable-tunnel: w33 -> [w66 _]
      disable-tunnel: [w67 w71] -> w37
      disable-tunnel: w36 -> [w67 w71]
      frame condition #0 {
        n100 = case shown="Default" w66 {
          selector: w66 -> [_ w68]
          frame "" {
          }
          frame Default {
            n101 = Concatenate Strings(w68, "Finished" ("string")) -> (w70:string)
            n102 = call <vilib>:"NI VeriStand - Print Debug String.vi"("Message"=w70) -> ()  [unwired: 10 in, 1 out]
          }
        }
      }
      frame condition #1 (active) {
      }
    }
    n103 = Tick Count (ms)() -> (millisecond timer value=w50:u32)
    n104 = feedback #1(w50) -> (w49:u32)
    n105 = Subtract(x=w50, y=w49) -> (x-y=w56:u32)
    n106 = Greater Or Equal?(x=w56, y=u32 1000) -> (x >= y?=w52:bool)
    n107 = case shown="True" w52 {
      tunnel: w37 -> [w72 w77]
      tunnel: [w73 w79] -> w51
      tunnel: w49 -> [w73 _]
      tunnel: w50 -> [_ w79]
      tunnel: w48 -> [_ w78]
      tunnel: [w72 w75] -> w45
      frame False {
      }
      frame True {
        n108 = call <vilib>:"TesterPresent.vi"("response required?"=FALSE, "diag ref in"=w78) -> ("error out"=w76:errorcluster)  [unwired: 7 in, 2 out]
        n109 = Merge Errors(w77, w76) -> (w75:errorcluster)
      }
    }
    n110 = feedback-in #1(w51) -> ()
    n111 = call "Global Stop Actions.vi"("Command"=Stop_Global_Commands."Read", "error in (no error)"=w45, "Stop on Error?"=FALSE, "vi reference"=w40) -> ("error out"=w44:errorcluster, "Latched Stop"=w43:bool)  [unwired: 5 in, 1 out]
    n112 = call "Report Error to Process.vi"("Error"=w44, "This VI"=w42) -> ()  [unwired: 10 in]
  }
  "error out" <- w16
